vi "Qalibrate_server.vi"(11 "RunExp 2":refnum<vi>) -> ()   [LabVIEW 2019]
uses:
  controls/GlobalExp.vi
  exp_status.vi
  Global.lvlib
panel:
  out "data out":string
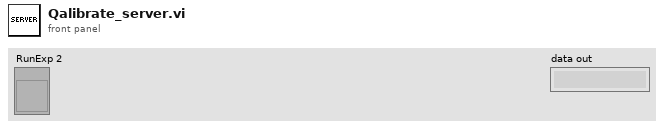
[diagram p1: front panel]
types:
  T1 = enum16{"Standard", "Buffered", "CRLF", "Immediate"}
  T2 = typedef "MasterExpControl.ctl" = cluster{"Main Steps":dbl, "Main Runs":dbl, "ExpStatus":enum16{"Innit", "Stop", "Idle", "MainRunning", "AuxRunning"}, "Main Current Step":dbl, "ExpNum":dbl, "NewData":bool, "date":string, "command":string, "Stop":bool, "Pause":bool, "Mathematica":string, "Main/Meta":bool, "UpdateMath":bool, "Camera":bool, "MetaExpOver":bool, "NextMetaExp":bool}
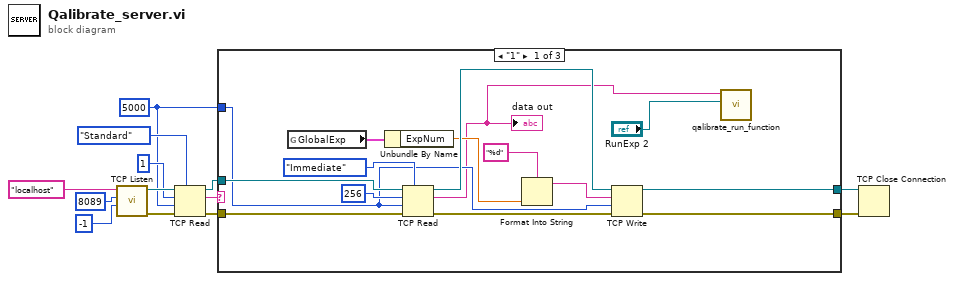
[diagram p0: block diagram]
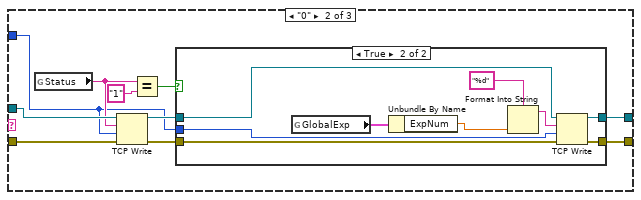
[diagram p2: hidden frame]
diagram:
  w1 = 5000 ("timeout ms (25000)")
  n1 = call <vilib>:"TCP Listen.vi"("timeout ms (wait forever: -1)"=-1, "port"=u16 8089, "service name"="localhost") -> ("error out"=w12:errorcluster, "connection ID"=w11:refnum<k5>)  [unwired: 4 in, 3 out]
  n2 = TCP Read(connection ID=w11, bytes to read=1, error in (no error)=w12, 7:T1."Standard" ("mode (standard)"), 9:w1) -> (connection ID out=w7:refnum<k5>, data out=w8:string, error out=w6:errorcluster)
  n3 = case shown="\"1\"" w8 {
    tunnel: w7 -> [w28 w38 w51]
    tunnel: w6 -> [w27 w37 w50]
    tunnel: [w23 w32 w51] -> w5
    tunnel: [w24 w31 w50] -> w4
    tunnel: w1 -> [w16 w29 _]
    frame "1" {
      n4 = global read "GlobalExp.vi" "GlobalExp"() -> (w20:T2)
      n5 = Unbundle By Name(w20) -> ("ExpNum"=w19:dbl)
      n6 = TCP Read(connection ID=w28, bytes to read=256, error in (no error)=w27, 7:T1."Immediate" ("mode (standard)"), 9:w16) -> (connection ID out=w26:refnum<k5>, data out=w15:string, error out=w25:errorcluster)
      "data out" <- w15
      n7 = Format Into String(format string="%d", w19) -> (resulting string=w17:string)  [unwired: 2 in, 1 out]
      n8 = TCP Write(connection ID=w26, data in=w17, error in (no error)=w25, 9:w16) -> (connection ID out=w23:refnum<k5>, error out=w24:errorcluster)  [unwired: 1 out]
      n9 = call "qalibrate_run_function.vi"("Run button ref"="RunExp 2", "function in"=w15) -> ()  [unwired: 10 in]
    }
    frame "0" {
      n10 = global read "exp_status.vi" "Status"() -> (w30:string)
      n11 = TCP Write(connection ID=w38, data in=w30, error in (no error)=w37, 9:w29) -> (connection ID out=w34:refnum<k5>, error out=w33:errorcluster)  [unwired: 1 out]
      n12 = Equal?(x=w30, y="1") -> (x = y?=w36:bool)
      n13 = case shown="True" w36 {
        tunnel: w34 -> [w40 w49]
        tunnel: w33 -> [w39 w48]
        tunnel: [w40 w47] -> w32
        tunnel: [w39 w46] -> w31
        tunnel: w29 -> [_ w41]
        frame False {
        }
        frame True {
          n14 = global read "GlobalExp.vi" "GlobalExp"() -> (w45:T2)
          n15 = Unbundle By Name(w45) -> ("ExpNum"=w44:dbl)
          n16 = Format Into String(format string="%d", w44) -> (resulting string=w42:string)  [unwired: 2 in, 1 out]
          n17 = TCP Write(connection ID=w49, data in=w42, error in (no error)=w48, 9:w41) -> (connection ID out=w47:refnum<k5>, error out=w46:errorcluster)  [unwired: 1 out]
        }
      }
    }
    frame "-1", Default {
    }
  }
  n18 = TCP Close Connection(connection ID=w5, error in (no error)=w4) -> ()  [unwired: 1 in, 2 out]
